vi "Read_WaterLevel.vi"() -> (0 "Meter":dbl(knob) scale=0.0..10.0, 1 "Waveform Chart":dbl(graph))   [LabVIEW 2024]
uses:
  <vilib>/DAQmx/read.llb/DAQmx Read (Analog DBL 1Chan 1Samp).vi
  <vilib>/DAQmx/create/channels.llb/DAQmx Create Channel (AI-Voltage-Basic).vi
  <vilib>/DAQmx/miscellaneous.llb/DAQmx Fill In Error Info.vi
panel:
  in  "stop":bool
  in  "DAQmx Physical Channel":tag
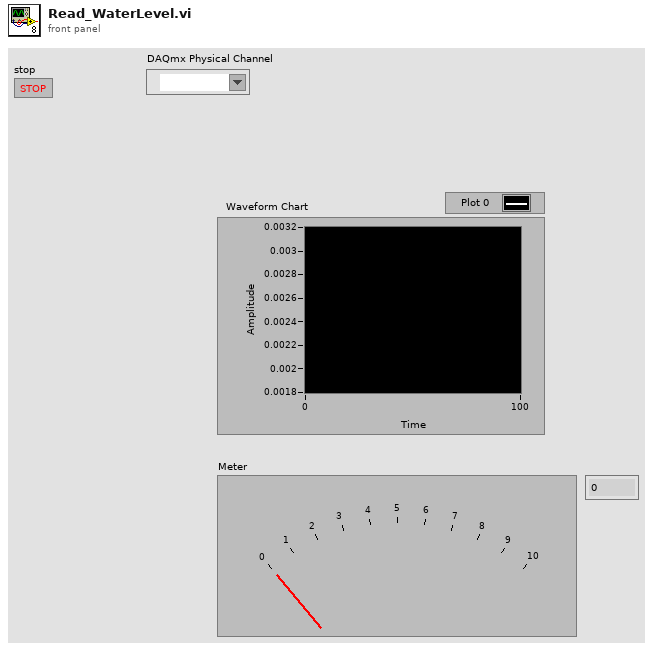
[diagram p1: front panel]
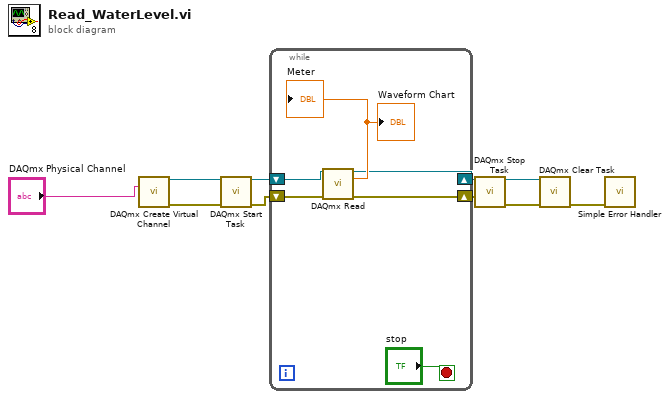
[diagram p0: block diagram]
diagram:
  n1 = call-poly <vilib>:"DAQmx Create Virtual Channel.vi"("physical channels"="DAQmx Physical Channel") -> ("task out"=w6:refnum<k21>, "error out"=w5:errorcluster)  [unwired: 13 in]
  n2 = call <vilib>:"DAQmx Start Task.vi"("task/channels in"=w6, "error in"=w5) -> ("task out"=w4:refnum<k21>, "error out"=w3:errorcluster)  [unwired: 12 in]
  n3 = while {
    shift-right: [w12] -> w1
    shift-left: w4 -> [w15]
    shift-right: [w13] -> w2
    shift-left: w3 -> [w14]
    stop <- "stop" stop-if-true
    n4 = call-poly <vilib>:"DAQmx Read.vi"("task/channels in"=w15, "error in"=w14) -> ("task out"=w12:refnum<k21>, "data"=→"Meter" →"Waveform Chart":dbl, "error out"=w13:errorcluster)  [unwired: 11 in]
  }
  n5 = call <vilib>:"DAQmx Stop Task.vi"("task/channels in"=w1, "error in"=w2) -> ("task out"=w9:refnum<k21>, "error out"=w8:errorcluster)  [unwired: 12 in]
  n6 = call <vilib>:"DAQmx Clear Task.vi"("task in"=w9, "error in"=w8) -> ("error out"=w10:errorcluster)  [unwired: 13 in]
  n7 = call <vilib>:"Simple Error Handler.vi"("error in (no error)"=w10) -> ()  [unwired: 4 in, 5 out]
